vi "Send LoadIntoSubPanel.vi"(7 "Message Priority (Normal)":T1=enum."Normal", 8 "error in (no error)":errorcluster, 10 "VI Refnum":refnum<vi>, 11 "Message Enqueuer":refnum<class "Message Enqueuer.lvclass">) -> (0 "error out":errorcluster, 3 "Message Enqueuer out":refnum<class "Message Enqueuer.lvclass">)   [LabVIEW 2020, in "ICameraTesting.lvlib" / "LoadIntoSubPanel Msg.lvclass"]
doc: "This VI sends the message to an actor."
uses:
  LoadIntoSubPanel Msg.lvclass
  LoadIntoSubPanel Msg.lvclass/LoadIntoSubPanel Msg.ctl
  <vilib>/ActorFramework/Message Enqueuer/Message Enqueuer.lvclass
  C:/Program Files (x86)/National Instruments/LabVIEW 2020/vi.lib/ActorFramework/Message/Message.lvclass
  E:/GitHub/Evaluation_Test/Labview/src/CameraTestingApp/ICameraTesting/ICameraTesting Messages/LoadIntoSubPanel Msg/LoadIntoSubPanel Msg.lvclass
  <vilib>/ActorFramework/Message Enqueuer/Message Priority.ctl
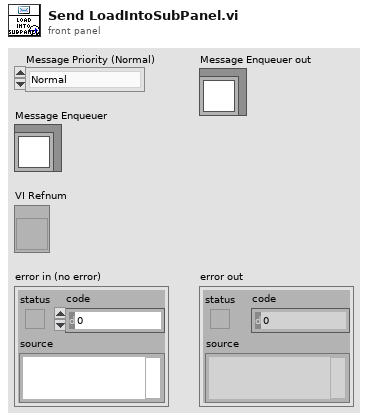
[diagram p1: front panel]
types:
  T1 = typedef "Actor Framework.lvlib/Message Enqueuer.lvclass/Message Priority.ctl" = enum16{"Low", "Normal", "High"}
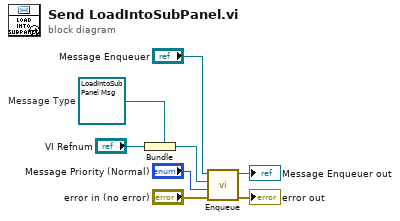
[diagram p0: block diagram]
diagram:
  w5 = refnum<class "LoadIntoSubPanel Msg.lvclass"> refnum  # Message Type
  n1 = Bundle(cluster=w5, "VI Refnum") -> (w4:refnum<class "LoadIntoSubPanel Msg.lvclass">)
  n2 = call <vilib>:"Enqueue.vi"("error in (no error)"="error in (no error)", "Message Priority (Normal)"="Message Priority (Normal)", "Message"=w4, "Message Enqueuer in"="Message Enqueuer") -> ("error out"=→"error out":errorcluster, "Message Enqueuer in"=→"Message Enqueuer out":refnum<class "Message Enqueuer.lvclass">)  [unwired: 6 in]
